vi "Compare Drivebase Curves.vi"() -> ()   [LabVIEW 2020]
uses:
  Robot Compare Info.ctl
  Motor Type.ctl
panel:
  in  "Remove":bool
  in  "Add":bool
  in  "Saved Compares":i32(listbox)
  in  "Compares":cluster{"Color":u32, "Info 2":T1}[](array[cluster])=[{"Color"=16716306, "Info 2"={"Motor Count"=4, "Motor Type"=enum."Neo", "Ratio"=0.09000000000000001, "Total Mass"=68.0388555, "Battery Voltage"=12.9, "Internal Resistance"=0.015, "Total Amps"=300.0}}, {"Color"=56321, "Info 2"={"Motor Count"=6, "Motor Type"=enum."Neo", "Ratio"=0.09000000000000001, "Total Mass"=68.0388555, "Battery Voltage"=12.9, "Internal Resistance"=0.015, "Total Amps"=300.0}}, {"Color"=2782463, "Info 2"={"Motor Count"=6, "Motor Type"=enum."CIM", "Ratio"=0.09, "Total Mass"=68.0388555, "Battery Voltage"=12.9, "Internal Resistance"=0.015, "Total Amps"=200.0}}, {"Color"=64255, "Info 2"={"Motor Count"=6, "Motor Type"=enum."miniCIM", "Ratio"=0.08, "Total Mass"=68.0388555, "Battery Voltage"=12.9, "Internal Resistance"=0.015, "Total Amps"=300.0}}, {"Color"=16776722, "Info 2"={"Motor Count"=4, "Motor Type"=enum."Falcon 500", "Ratio"=0.09, "Total Mass"=68.0388555, "Battery Voltage"=12.9, "Internal Resistance"=0.015, "Total Amps"=300.0}}] {"Info 2"."Internal Resistance" min=0.0 step=0.005 format="%#_13g"; "Info 2"."Battery Voltage" min=6.0 format="%#_13g"; "Info 2"."Total Mass" min=0.0 step=2.2679618500000003; "Info 2"."Total Amps" min=0.0 step=20.0 format="%#_13g"; "Info 2"."Ratio" min=0.005 step=0.01; "Info 2"."Motor Count" min=2 step=2}
  out "Accel vs Distance for T seconds":T3(graph)
  in  "Sprint Time":dbl[unit](slide)=1.0 scale=0.0..5.0 scale format="%#_2g"
  out "Speed vs Distance for T seconds":T4(graph)
  # "Assumes a 6\" wheel"
  # "Neo + SparkMax\n1.15 lbs, $125\n\n4x 4.6lbs & $500\n6x 6.9 lbs & $750"
  # "Neo 550 + SparkMax\n.31 lbs, $105\n\n6x 1.86 lbs & $630"
  # "Falcon 500\n1.1 lbs, $140\n\n4x 4.4lbs & $560"
  # "CIM + Victor SPX\n3.06 lbs, $83\n\n6x 18.36 lbs & $498"
  # "miniCIM + Victor SPX\n2.36 lbs, $80\n\n6x 14.16 lbs & $480"
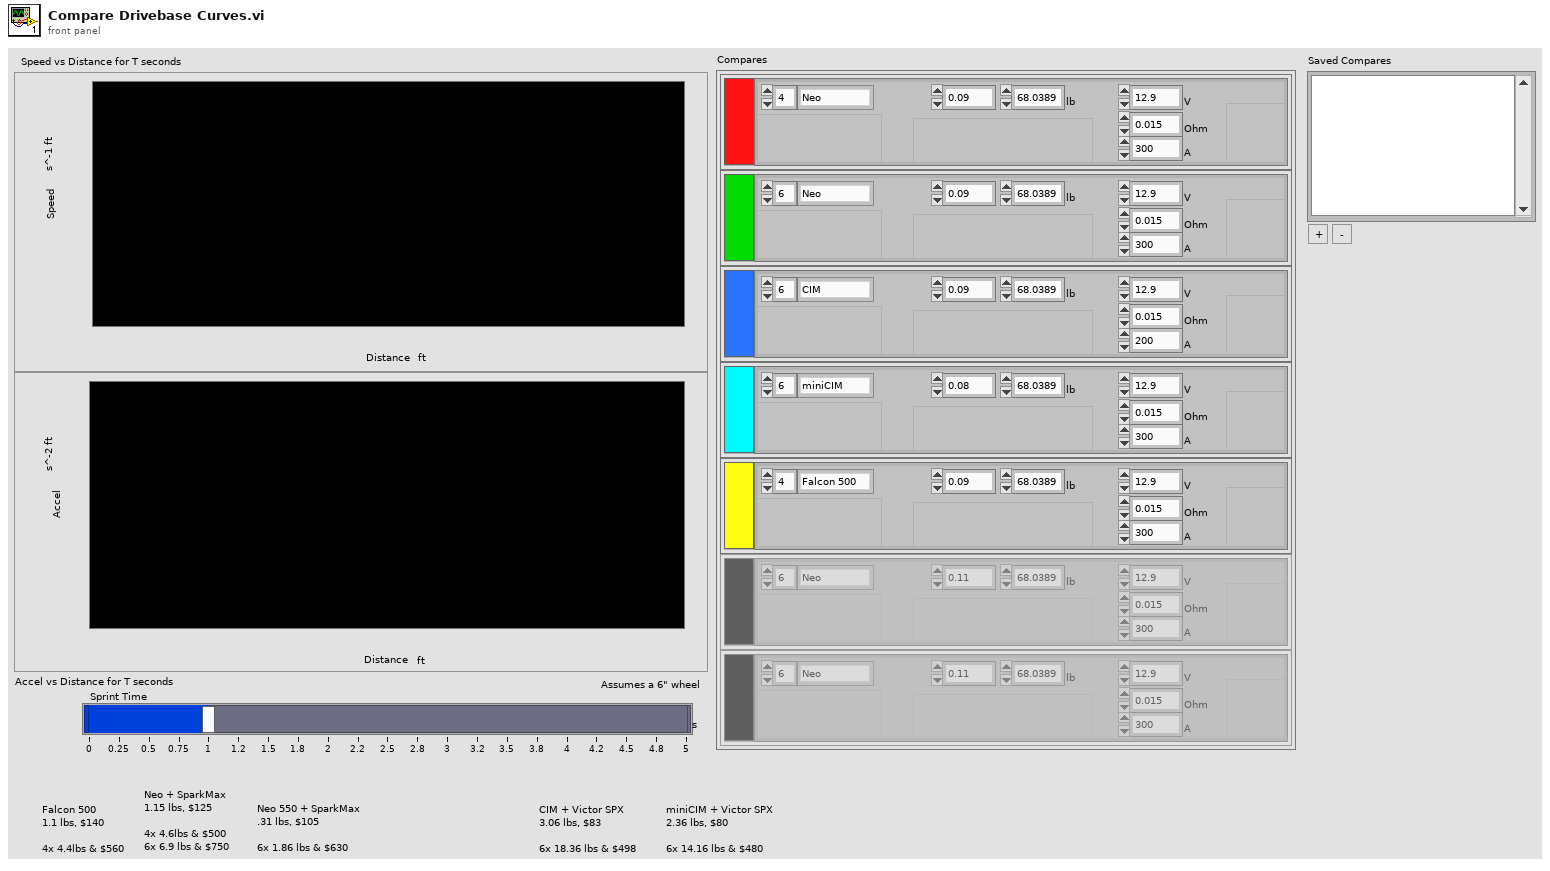
[diagram p1: front panel]
types:
  T1 = typedef "Robot Compare Info.ctl" = cluster{"Motor Count":i32, "Motor Type":T2, "Ratio":dbl, "Total Mass":dbl[unit], "Battery Voltage":dbl[unit], "Internal Resistance":dbl[unit], "Total Amps":dbl[unit]}
  T2 = typedef "Motor Type.ctl" = enum16{"Custom", "775 pro", "CIM", "miniCIM", "Neo", "Neo 550", "Falcon 500"}
  T3 = cluster{cluster{"Distance":dbl[unit], "Accel":dbl[unit]}[]}[]
  T4 = cluster{cluster{"Distance":dbl[unit], "Velocity":dbl[unit]}[]}[]
  T5 = cluster{"Name":string, "Color":u32, "Style":i32, "Point Style":i32, "Name Visible":bool, "Allow Drag":bool, "Cursor Mode":i32, "Plot":i32, "Index":i32, "Position":cluster{"X":dbl, "Y":dbl}, "X Scale":u32, "Y Scale":u32, "Watch Plots":i32[], "Watch All Plots":bool, "Plot Area":i32, "Label Offset":cluster{"X":dbl, "Y":dbl}}
  T6 = cluster{"Color":u32, "Array":cluster{dbl[unit], cluster{"Distance":dbl[unit], "Accel":dbl[unit], "Velocity":dbl[unit]}}[]}[]
  T7 = enum8{"Enabled", "Disabled", "Disabled and Grayed Out"}
  T8 = cluster{"Color":u32, "Array":cluster{dbl[unit], cluster{"Distance":dbl[unit], "Accel":dbl[unit], "Velocity":dbl[unit]}}[]}
  T9 = cluster{"Battery Voltage":dbl[unit], "Internal Resistance":dbl[unit], "Total Amps":dbl[unit]}
  T10 = cluster{dbl[unit], cluster{"Distance":dbl[unit], "Accel":dbl[unit], "Velocity":dbl[unit]}}[]
  T11 = cluster{"Distance":dbl[unit], "Accel":dbl[unit], "Velocity":dbl[unit]}
  T12 = cluster{"Distance":dbl[unit], "Velocity":dbl[unit]}
  T13 = cluster{cluster{"Distance":dbl[unit], "Accel":dbl[unit]}[]}
  T14 = cluster{cluster{"Distance":dbl[unit], "Velocity":dbl[unit]}[]}
  T15 = typedef "LVPoint32TypeDef.ctl" = cluster{"Horizontal":i32, "Vertical":i32}
  T16 = typedef "LVRectTypeDef.ctl" = cluster{"Left":i16, "Top":i16, "Right":i16, "Bottom":i16}
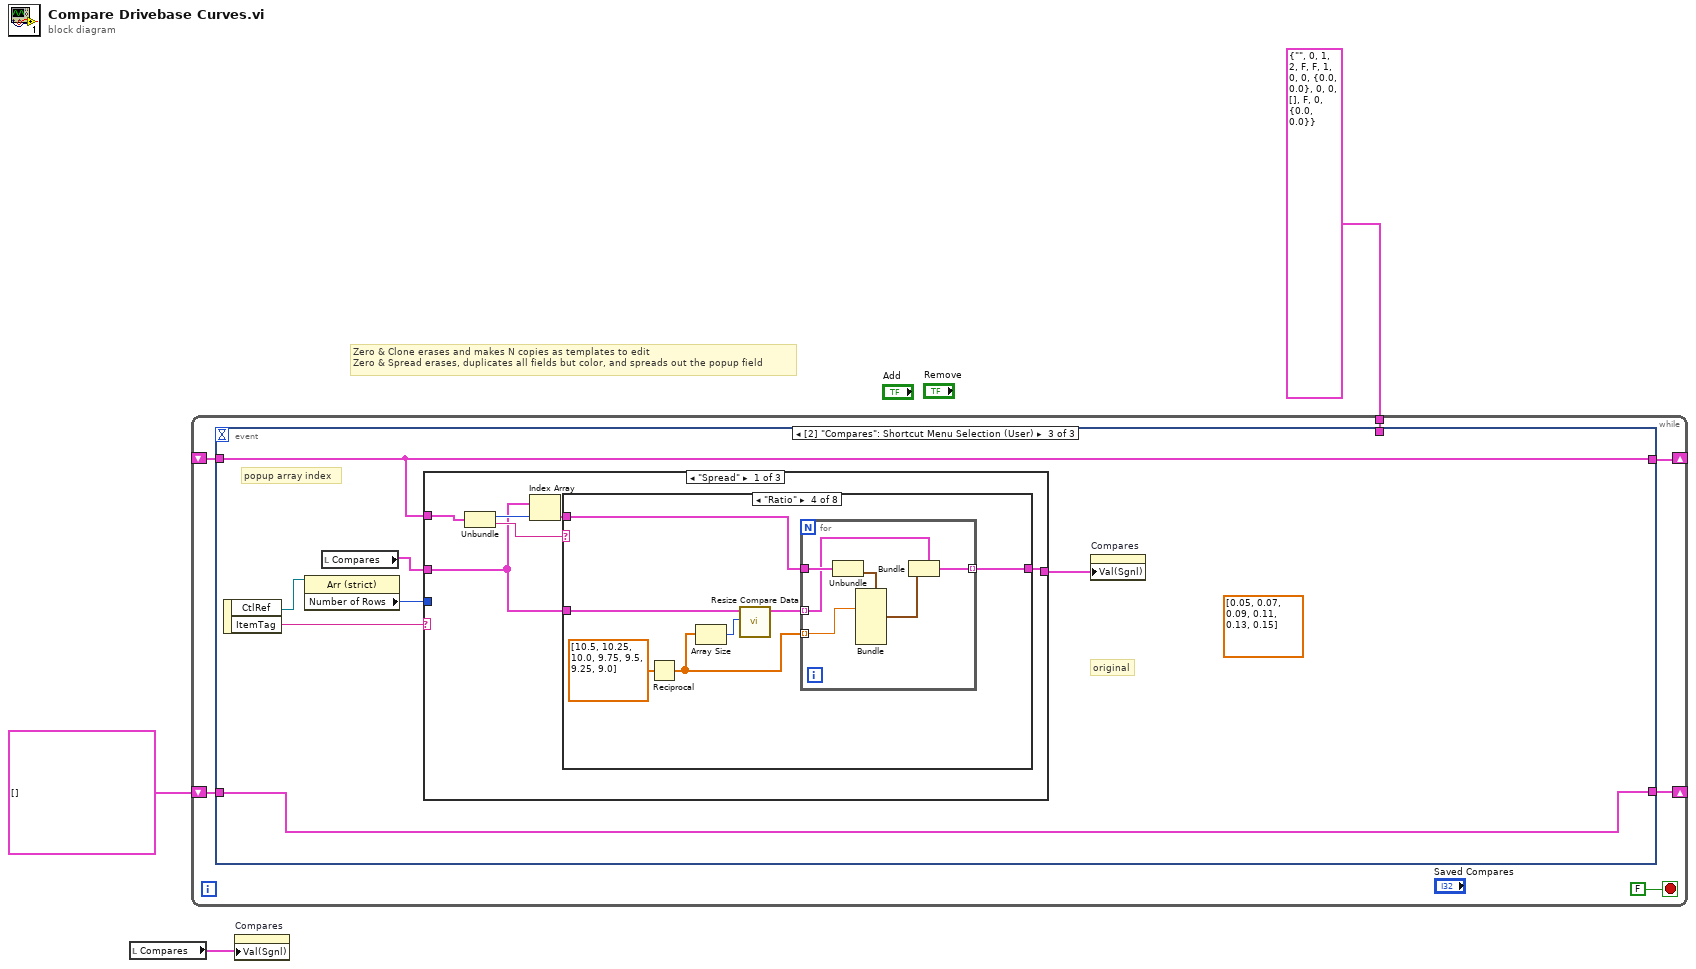
[diagram p0: block diagram]
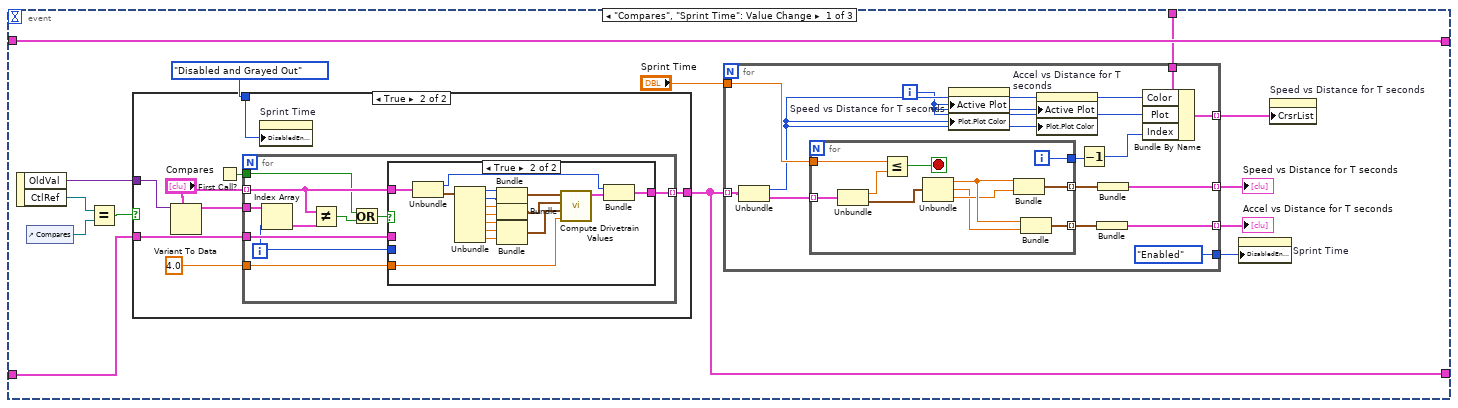
[diagram p2: hidden frame]
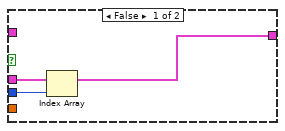
[diagram p4: hidden frame]
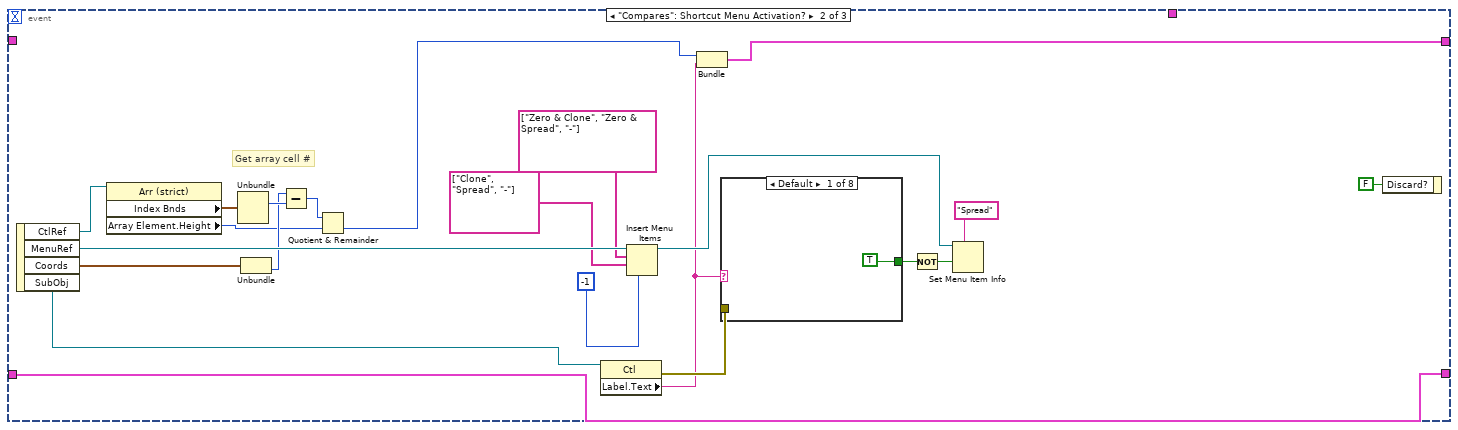
[diagram p5: hidden frame]
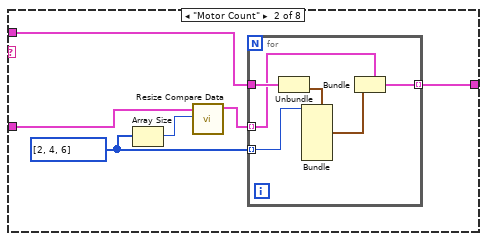
[diagram p14: hidden frame]
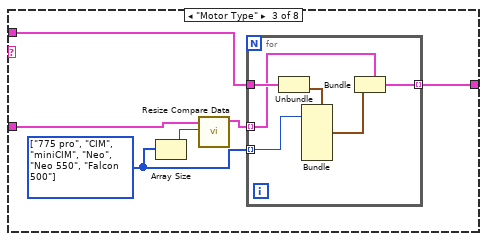
[diagram p15: hidden frame]
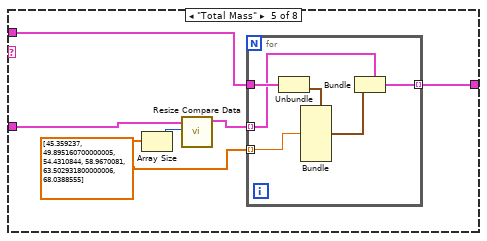
[diagram p16: hidden frame]
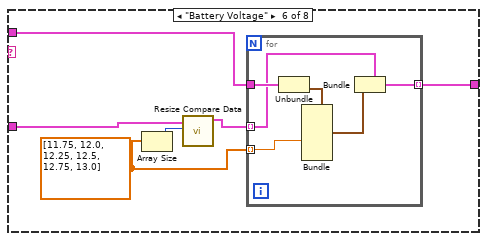
[diagram p17: hidden frame]
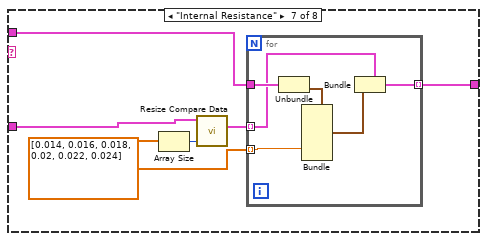
[diagram p18: hidden frame]
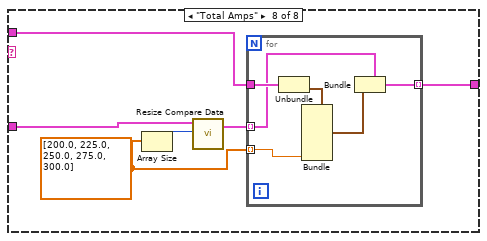
[diagram p19: hidden frame]
diagram:
  # "Zero & Clone erases and makes N copies as templates to edit\nZero & Spread erases, duplicates all fields but color, and spreads out the popup field"
  n1 = local read "Compares"() -> (w3:cluster{"Color":u32, "Info 2":T1}[])
  n2 = while {
    shift-right: [w8] -> _
    shift-left: T6 [] -> [w7]
    shift-right: [w6] -> _
    shift-left: _ -> [w5]
    tunnel: T5 {"Name"="", "Color"=0, "Style"=1, "Point Style"=2, "Name Visible"=FALSE, "Allow Drag"=FALSE, "Cursor Mode"=1, "Plot"=0, "Index"=0, "Position"={"X"=0.0, "Y"=0.0}, "X Scale"=0, "Y Scale"=0, "Watch Plots"=[], "Watch All Plots"=FALSE, "Plot Area"=0, "Label Offset"={"X"=0.0, "Y"=0.0}} -> [w4]
    stop <- FALSE stop-if-true
    n3 = event shown="[2] \"Compares\": Shortcut Menu Selection (User)" {
      selector: _ -> [_ _ _]
      dyn-events: _ -> [_ _ _]
      timeout: _ -> [_ _ _]
      tunnel: [w21 w87 w110] -> w8
      tunnel: w7 -> [w17 w87 w110]
      tunnel: [w12 w91 w113] -> w6
      tunnel: w5 -> [w12 _ w113]
      tunnel: w4 -> [w11 _ _]
      event "Compares", "Sprint Time": Value Change {
        n4 = event-data() -> ("OldVal"=w15:variant, "CtlRef"=w19:refnum<vi>)  [unwired: 1 in]
        n5 = control-ref of="Compares"() -> (w20:refnum<vi>)
        n6 = Equal?(x=w19, y=w20) -> (x = y?=w18:bool)
        n7 = case shown="True" w18 {
          tunnel: [w24 w32] -> w21
          tunnel: w17 -> [w24 w27]
          tunnel: w15 -> [_ w30]
          tunnel: T7."Disabled and Grayed Out" ("Disabled") -> [_ w25]
          frame False {
          }
          frame True {
            n8 = Variant To Data(type="Compares", Variant=w30) -> (data=w28:cluster{"Color":u32, "Info 2":T1}[])  [unwired: 1 in, 1 out]
            n9 = First Call?() -> (First Call?: T/F=w26:bool)
            n10 = for {
              tunnel: dbl[unit] 4.0 ("Sprint Time") -> [w42]
              tunnel: [w41] -> w32 mode=indexing
              tunnel: "Compares" -> [w40] mode=indexing
              tunnel: w28 -> [w37]
              tunnel: w27 -> [w38]
              tunnel: w26 -> [w33]
              i -> [w35]
              # "Vary info"
              n11 = Index Array(array=w37, index=w35) -> (element=w36:cluster{"Color":u32, "Info 2":T1})
              n12 = Not Equal?(x=w40, y=w36) -> (x != y?=w39:bool)
              n13 = Or(x=w33, y=w39) -> (x .or. y?=w34:bool)
              n14 = case shown="True" w34 {
                tunnel: w42 -> [_ w61]
                tunnel: [w44 w59] -> w41
                tunnel: w40 -> [_ w58]
                tunnel: w38 -> [w45 _]
                tunnel: w35 -> [w43 _]
                frame False {
                  n15 = Index Array(array=w45, index=w43) -> (element=w44:T8)
                }
                frame True {
                  n16 = Unbundle(w58) -> ("Color"=w46:u32, "Info 2"=w57:T1)
                  n17 = Unbundle(w57) -> ("Motor Count"=w56:i32, "Motor Type"=w55:T2, "Ratio"=w53:dbl, "Total Mass"=w52:dbl[unit], "Battery Voltage"=w50:dbl[unit], "Internal Resistance"=w49:dbl[unit], "Total Amps"=w48:dbl[unit])
                  n18 = Bundle("Motor Count"=w56, "Motor Type"=w55) -> (w54:cluster{"Motor Count":i32, "Motor Type":T2})  [unwired: 1 in]
                  n19 = Bundle("Ratio"=w53, "Total Mass"=w52) -> (w51:cluster{"Ratio":dbl, "Total Mass":dbl[unit]})  [unwired: 1 in]
                  n20 = Bundle("Battery Voltage"=w50, "Internal Resistance"=w49, "Total Amps"=w48) -> (w47:T9)  [unwired: 1 in]
                  n21 = call "Compute Drivetrain Values.vi"("Motor count & type"=w54, "ratio & mass"=w51, "Battery Info"=w47, "Loop Time"=w61) -> ("Array"=w60:T10)  [unwired: 6 in]
                  n22 = Bundle("Color"=w46, "Array"=w60) -> (w59:T8)  [unwired: 1 in]
                }
              }
            }
            n23 = property on="Sprint Time" class="Slide (strict)"("DisabledEnum"=w25) -> ()  [unwired: 2 in, 2 out]
          }
        }
        n24 = for {
          tunnel: w21 -> [w75] mode=indexing
          tunnel: [w72] -> w23 mode=indexing
          tunnel: [w70] -> w22 mode=indexing
          tunnel: "Sprint Time" -> [w69]
          tunnel: [T7."Enabled" ("Disabled")] -> w13
          tunnel: w11 -> [w67]
          tunnel: [w66] -> w10 mode=indexing
          i -> [w64]
          n25 = Unbundle(w75) -> ("Color"=w65:u32, "Array"=w74:T10)
          n26 = for {
            tunnel: w74 -> [w86] mode=indexing
            tunnel: [w77] -> w73 mode=indexing
            tunnel: [w84] -> w71 mode=indexing
            tunnel: w69 -> [w79]
            tunnel: [w76] -> w63
            i -> [w76]
            stop <- w78 stop-if-true
            n27 = Unbundle(w86) -> (w80:dbl[unit], w85:T11)
            n28 = Less Or Equal?(x=w79, y=w80) -> (x <= y?=w78:bool)
            n29 = Unbundle(w85) -> ("Distance"=w83:dbl[unit], "Accel"=w81:dbl[unit], "Velocity"=w82:dbl[unit])
            n30 = Bundle("Distance"=w83, "Velocity"=w82) -> (w77:T12)  [unwired: 1 in]
            n31 = Bundle("Distance"=w83, "Accel"=w81) -> (w84:cluster{"Distance":dbl[unit], "Accel":dbl[unit]})  [unwired: 1 in]
          }
          n32 = property on="Speed vs Distance for T seconds" class="XYGraph (strict)"("Active Plot"=w64, "Plot.Plot Color"=w65) -> ()  [unwired: 2 in, 2 out]
          n33 = property on="Accel vs Distance for T seconds" class="XYGraph (strict)"("Active Plot"=w64, "Plot.Plot Color"=w65) -> ()  [unwired: 2 in, 2 out]
          n34 = Decrement(x=w63) -> (x-1=w62:i32)
          n35 = Bundle(w71) -> (w70:T13)  [unwired: 1 in]
          n36 = Bundle(w73) -> (w72:T14)  [unwired: 1 in]
          n37 = Bundle By Name(cluster=w67, "Color"=w65, "Plot"=w64, "Index"=w62) -> (w66:T5)
        }
        "Speed vs Distance for T seconds" <- w23
        "Accel vs Distance for T seconds" <- w22
        n38 = property on="Sprint Time" class="Slide (strict)"("DisabledEnum"=w13) -> ()  [unwired: 2 in, 2 out]
        n39 = property on="Speed vs Distance for T seconds" class="XYGraph (strict)"("CrsrList"=w10) -> ()  [unwired: 2 in, 2 out]
      }
      event "Compares": Shortcut Menu Activation? {
        # "Get array cell #"
        n40 = event-data() -> ("CtlRef"=w99:refnum<vi>, "MenuRef"=w108:refnum<k9>, "Coords"=w98:T15, "SubObj"=w105:refnum<vi>)  [unwired: 1 in]
        n41 = property class="Arr (strict)"(reference=w99) -> ("Index Bnds"=w97:T16, "Array Element.Height"=w93:u32)  [unwired: 1 in, 2 out]
        n42 = Unbundle(w97) -> ("Top"=w96:i16)  [unwired: 3 out]
        n43 = Unbundle(w98) -> ("Vertical"=w95:i32)  [unwired: 1 out]
        n44 = Subtract(x=w95, y=w96) -> (x-y=w94:i32)
        n45 = Quotient & Remainder(x=w94, y=w93) -> (floor(x/y)=w92:u32)  [unwired: 1 out]
        n46 = property class="Ctl"(reference=w105) -> (error out=w89:errorcluster, "Label.Text"=w88:string)  [unwired: 1 in, 1 out]
        n47 = Insert Menu Items(4:-1, 7:string[] ["Clone", "Spread", "-"] ("item names"), 8:string[] ["Zero & Clone", "Zero & Spread", "-"] ("item names"), 9:w108) -> (3:w104:refnum<k9>)  [unwired: 2 in, 2 out]
        n48 = Bundle(w92, "Label.Text"=w88) -> (w91:cluster{u32, "Label.Text":string})  [unwired: 1 in]
        n49 = case shown="Default" w88 {
          tunnel: [TRUE _ _ _ _ _ _ _] -> w102
          tunnel: w89 -> [_ _ _ _ _ _ _ _]
          frame Default {
          }
          frame "Motor Count" {
          }
          frame "Motor Type" {
          }
          frame "Ratio" {
          }
          frame "Total Mass" {
          }
          frame "Battery Voltage" {
          }
          frame "Internal Resistance" {
          }
          frame "Total Amps" {
          }
        }
        n50 = Not(x=w102) -> (.not. x?=w101:bool)
        n51 = Set Menu Item Info(7:"Spread", 9:w101, 11:w104) -> ()  [unwired: 4 in, 2 out]
        n52 = event-data("Discard?"=FALSE) -> ()  [unwired: 1 in, 1 out]
      }
      event "Compares": Shortcut Menu Selection (User) {
        (unwired) dbl[] [0.05, 0.07, 0.09, 0.11, 0.13, 0.15]
        # "original"
        # "popup array index"
        n53 = event-data() -> ("CtlRef"=w115:refnum<vi>, "ItemTag"=w116:string)  [unwired: 1 in]
        n54 = property class="Arr (strict)"(reference=w115) -> ("Number of Rows"=w114:u32)  [unwired: 1 in, 2 out]
        n55 = local read "Compares"() -> (w112:cluster{"Color":u32, "Info 2":T1}[])
        n56 = case shown="\"Spread\"" w116 {
          tunnel: w114 -> [_ _ _]
          tunnel: w113 -> [w122 _ w211]
          tunnel: w112 -> [w118 w209 w213]
          tunnel: [w117 w209 w212] -> w111
          frame "Spread" {
            n57 = Unbundle(w122) -> (w121:u32, "Label.Text"=w120:string)
            n58 = Index Array(array=w118, index=w121) -> (element=w119:cluster{"Color":u32, "Info 2":T1})
            n59 = case shown="\"Ratio\"" w120 {
              tunnel: w119 -> [_ w129 w141 w154 w166 w178 w190 w202]
              tunnel: w118 -> [w123 w126 w138 w151 w162 w175 w186 w198]
              tunnel: [w123 w128 w140 w153 w165 w177 w189 w201] -> w117
              frame Default {
              }
              frame "Motor Count" {
                w127 = i32[] [2, 4, 6]
                n60 = Array Size(array=w127) -> (size(s)=w124:i32)
                n61 = call "Resize Compare Data.vi"("Size"=w124, "Compares in"=w126) -> ("Compares out"=w125:cluster{"Color":u32, "Info 2":T1}[])  [unwired: 9 in]
                n62 = for {
                  tunnel: w125 -> [w133] mode=indexing
                  tunnel: w129 -> [w135]
                  tunnel: w127 -> [w131] mode=indexing
                  tunnel: [w130] -> w128 mode=indexing
                  n63 = Unbundle(w135) -> ("Info 2"=w134:T1)  [unwired: 1 out]
                  n64 = Bundle(cluster=w134, "Motor Count"=w131) -> (w132:T1)  [unwired: 6 in]
                  n65 = Bundle(cluster=w133, "Info 2"=w132) -> (w130:cluster{"Color":u32, "Info 2":T1})  [unwired: 1 in]
                }
              }
              frame "Motor Type" {
                w139 = T2[] [enum."775 pro", enum."CIM", enum."miniCIM", enum."Neo", enum."Neo 550", enum."Falcon 500"] items=["Custom", "775 pro", "CIM", "miniCIM", "Neo", "Neo 550", "Falcon 500"]
                n66 = Array Size(array=w139) -> (size(s)=w136:i32)
                n67 = call "Resize Compare Data.vi"("Size"=w136, "Compares in"=w138) -> ("Compares out"=w137:cluster{"Color":u32, "Info 2":T1}[])  [unwired: 9 in]
                n68 = for {
                  tunnel: w137 -> [w145] mode=indexing
                  tunnel: w141 -> [w147]
                  tunnel: w139 -> [w142] mode=indexing
                  tunnel: [w143] -> w140 mode=indexing
                  n69 = Unbundle(w147) -> ("Info 2"=w146:T1)  [unwired: 1 out]
                  n70 = Bundle(cluster=w146, "Motor Type"=w142) -> (w144:T1)  [unwired: 6 in]
                  n71 = Bundle(cluster=w145, "Info 2"=w144) -> (w143:cluster{"Color":u32, "Info 2":T1})  [unwired: 1 in]
                }
              }
              frame "Ratio" {
                n72 = Reciprocal(x=dbl[] [10.5, 10.25, 10.0, 9.75, 9.5, 9.25, 9.0]) -> (1/x=w148:dbl[])
                n73 = Array Size(array=w148) -> (size(s)=w152:i32)
                n74 = call "Resize Compare Data.vi"("Size"=w152, "Compares in"=w151) -> ("Compares out"=w150:cluster{"Color":u32, "Info 2":T1}[])  [unwired: 9 in]
                n75 = for {
                  tunnel: w150 -> [w158] mode=indexing
                  tunnel: w154 -> [w160]
                  tunnel: w148 -> [w155] mode=indexing
                  tunnel: [w156] -> w153 mode=indexing
                  n76 = Unbundle(w160) -> ("Info 2"=w159:T1)  [unwired: 1 out]
                  n77 = Bundle(cluster=w159, "Ratio"=w155) -> (w157:T1)  [unwired: 6 in]
                  n78 = Bundle(cluster=w158, "Info 2"=w157) -> (w156:cluster{"Color":u32, "Info 2":T1})  [unwired: 1 in]
                }
              }
              frame "Total Mass" {
                w164 = dbl[unit][] [45.359237, 49.895160700000005, 54.4310844, 58.9670081, 63.502931800000006, 68.0388555]
                n79 = Array Size(array=w164) -> (size(s)=w163:i32)
                n80 = call "Resize Compare Data.vi"("Size"=w163, "Compares in"=w162) -> ("Compares out"=w161:cluster{"Color":u32, "Info 2":T1}[])  [unwired: 9 in]
                n81 = for {
                  tunnel: w161 -> [w170] mode=indexing
                  tunnel: w166 -> [w172]
                  tunnel: w164 -> [w167] mode=indexing
                  tunnel: [w168] -> w165 mode=indexing
                  n82 = Unbundle(w172) -> ("Info 2"=w171:T1)  [unwired: 1 out]
                  n83 = Bundle(cluster=w171, "Total Mass"=w167) -> (w169:T1)  [unwired: 6 in]
                  n84 = Bundle(cluster=w170, "Info 2"=w169) -> (w168:cluster{"Color":u32, "Info 2":T1})  [unwired: 1 in]
                }
              }
              frame "Battery Voltage" {
                w176 = dbl[unit][] [11.75, 12.0, 12.25, 12.5, 12.75, 13.0]
                n85 = Array Size(array=w176) -> (size(s)=w174:i32)
                n86 = call "Resize Compare Data.vi"("Size"=w174, "Compares in"=w175) -> ("Compares out"=w173:cluster{"Color":u32, "Info 2":T1}[])  [unwired: 9 in]
                n87 = for {
                  tunnel: w173 -> [w182] mode=indexing
                  tunnel: w178 -> [w184]
                  tunnel: w176 -> [w179] mode=indexing
                  tunnel: [w180] -> w177 mode=indexing
                  n88 = Unbundle(w184) -> ("Info 2"=w183:T1)  [unwired: 1 out]
                  n89 = Bundle(cluster=w183, "Battery Voltage"=w179) -> (w181:T1)  [unwired: 6 in]
                  n90 = Bundle(cluster=w182, "Info 2"=w181) -> (w180:cluster{"Color":u32, "Info 2":T1})  [unwired: 1 in]
                }
              }
              frame "Internal Resistance" {
                w188 = dbl[unit][] [0.014, 0.016, 0.018, 0.02, 0.022, 0.024]
                n91 = Array Size(array=w188) -> (size(s)=w185:i32)
                n92 = call "Resize Compare Data.vi"("Size"=w185, "Compares in"=w186) -> ("Compares out"=w187:cluster{"Color":u32, "Info 2":T1}[])  [unwired: 9 in]
                n93 = for {
                  tunnel: w187 -> [w194] mode=indexing
                  tunnel: w190 -> [w196]
                  tunnel: w188 -> [w191] mode=indexing
                  tunnel: [w192] -> w189 mode=indexing
                  n94 = Unbundle(w196) -> ("Info 2"=w195:T1)  [unwired: 1 out]
                  n95 = Bundle(cluster=w195, "Internal Resistance"=w191) -> (w193:T1)  [unwired: 6 in]
                  n96 = Bundle(cluster=w194, "Info 2"=w193) -> (w192:cluster{"Color":u32, "Info 2":T1})  [unwired: 1 in]
                }
              }
              frame "Total Amps" {
                w200 = dbl[unit][] [200.0, 225.0, 250.0, 275.0, 300.0]
                n97 = Array Size(array=w200) -> (size(s)=w199:i32)
                n98 = call "Resize Compare Data.vi"("Size"=w199, "Compares in"=w198) -> ("Compares out"=w197:cluster{"Color":u32, "Info 2":T1}[])  [unwired: 9 in]
                n99 = for {
                  tunnel: w197 -> [w206] mode=indexing
                  tunnel: w202 -> [w208]
                  tunnel: w200 -> [w203] mode=indexing
                  tunnel: [w204] -> w201 mode=indexing
                  n100 = Unbundle(w208) -> ("Info 2"=w207:T1)  [unwired: 1 out]
                  n101 = Bundle(cluster=w207, "Total Amps"=w203) -> (w205:T1)  [unwired: 6 in]
                  n102 = Bundle(cluster=w206, "Info 2"=w205) -> (w204:cluster{"Color":u32, "Info 2":T1})  [unwired: 1 in]
                }
              }
            }
          }
          frame Default {
          }
          frame "Clone" {
            n103 = Unbundle(w211) -> (w210:u32)  [unwired: 1 out]
            n104 = Index Array(array=w213, index=w210) -> (element=w214:cluster{"Color":u32, "Info 2":T1})
            n105 = for {
              tunnel: w213 -> [w219] mode=indexing
              tunnel: w214 -> [w218]
              tunnel: [w215] -> w212 mode=indexing
              n106 = Unbundle(w219) -> ("Color"=w217:u32)  [unwired: 1 out]
              n107 = Unbundle(w218) -> ("Info 2"=w216:T1)  [unwired: 1 out]
              n108 = Bundle("Color"=w217, "Info 2"=w216) -> (w215:cluster{"Color":u32, "Info 2":T1})  [unwired: 1 in]
            }
          }
        }
        n109 = property on="Compares" class="Arr (strict)"("Val(Sgnl)"=w111) -> ()  [unwired: 2 in, 2 out]
      }
    }
  }
  n110 = property on="Compares" class="Arr (strict)"("Val(Sgnl)"=w3) -> ()  [unwired: 2 in, 2 out]
